vi "prediction bounds.vi"(6 "damping":dbl, 7 "amplitude":dbl, 8 "error in (no error)":errorcluster, 9 "Hours array":dbl[](array[numeric]), 10 "Previous Hours Array":dbl[](array[numeric]), 11 "Previous Data Array":dbl[](array[numeric])) -> (0 "error out":errorcluster, 2 "Lower Bound":cluster{"Hours array":dbl[], "P(A)":dbl[]}, 3 "Upper Bound":cluster{"Hours array":dbl[], "P(A)":dbl[]})   [LabVIEW 2014, in "Data Trends.lvlib"]
uses:
  Data Trends.lvlib
  <vilib>/Analysis/6fits.llb/Prediction Interval (Exp).vi
  <vilib>/Analysis/polynomials.llb/1D Polynomial Evaluation (DBL).vi
  <vilib>/Analysis/NI_AALPro.lvlib
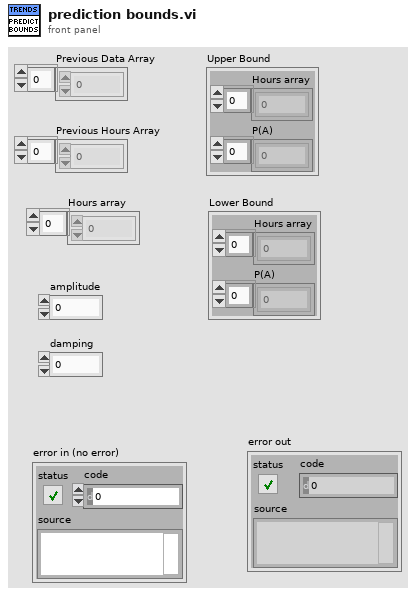
[diagram p1: front panel]
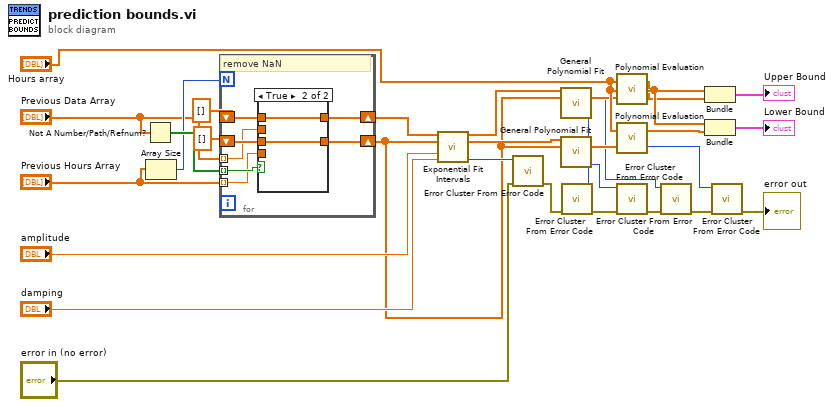
[diagram p0: block diagram]
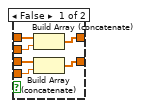
[diagram p2: hidden frame]
diagram:
  n1 = Not A Number/Path/Refnum?(number/path/refnum="Previous Data Array") -> (NaN/Path/Refnum?=w10:bool[])
  n2 = Array Size(array="Previous Hours Array") -> (size(s)=w9:i32)
  n3 = for {
    N: w9 -> [_]
    tunnel: w10 -> [w37] mode=indexing
    shift-right: [w36] -> w3
    shift-left: dbl[] [] -> [w35]
    shift-right: [w34] -> w6
    shift-left: dbl[] [] -> [w33]
    tunnel: "Previous Hours Array" -> [w32] mode=indexing
    tunnel: "Previous Data Array" -> [w31] mode=indexing
    # "remove NaN"
    n4 = case shown="True" w37 {
      tunnel: [w42 w45] -> w36
      tunnel: w35 -> [w43 w45]
      tunnel: [w41 w44] -> w34
      tunnel: w33 -> [w40 w44]
      tunnel: w32 -> [w39 _]
      tunnel: w31 -> [w38 _]
      frame False {
        n5 = Build Array (concatenate)(w40, w38) -> (w41:dbl[])
        n6 = Build Array (concatenate)(w43, w39) -> (w42:dbl[])
      }
      frame True {
      }
    }
  }
  n7 = call-poly <vilib>:"Exponential Fit Intervals.vi"("Y"=w6, "X"=w3, "amplitude"="amplitude", "damping"="damping") -> ("Upper Bound"=w26:dbl[], "Lower Bound"=w24:dbl[], "error"=w21:i32)  [unwired: 9 in]
  n8 = call <vilib>:"Error Cluster From Error Code.vi"("error in (no error)"="error in (no error)", "error code (0)"=w21) -> ("error out"=w19:errorcluster)  [unwired: 7 in]
  n9 = call <vilib>:"General Polynomial Fit.vi"("Y"=w26, "X"=w3) -> ("Polynomial Coefficients"=w28:dbl[], "error"=w16:i32)  [unwired: 10 in, 2 out]
  n10 = call <vilib>:"General Polynomial Fit.vi"("Y"=w24, "X"=w3) -> ("Polynomial Coefficients"=w25:dbl[], "error"=w15:i32)  [unwired: 10 in, 2 out]
  n11 = call <vilib>:"Error Cluster From Error Code.vi"("error in (no error)"=w19, "error code (0)"=w16) -> ("error out"=w18:errorcluster)  [unwired: 7 in]
  n12 = call-poly <vilib>:"Polynomial Evaluation.vi"("P(x)"=w28, "A"="Hours array") -> ("error"=w14:i32, "P(A)"=w2:dbl[])
  n13 = call-poly <vilib>:"Polynomial Evaluation.vi"("P(x)"=w25, "A"="Hours array") -> ("error"=w12:i32, "P(A)"=w1:dbl[])
  n14 = call <vilib>:"Error Cluster From Error Code.vi"("error in (no error)"=w18, "error code (0)"=w15) -> ("error out"=w17:errorcluster)  [unwired: 7 in]
  n15 = call <vilib>:"Error Cluster From Error Code.vi"("error in (no error)"=w17, "error code (0)"=w14) -> ("error out"=w13:errorcluster)  [unwired: 7 in]
  n16 = Bundle("Hours array"="Hours array", "P(A)"=w2) -> (→"Upper Bound":cluster{"Hours array":dbl[], "P(A)":dbl[]})  [unwired: 1 in]
  n17 = Bundle("Hours array"="Hours array", "P(A)"=w1) -> (→"Lower Bound":cluster{"Hours array":dbl[], "P(A)":dbl[]})  [unwired: 1 in]
  n18 = call <vilib>:"Error Cluster From Error Code.vi"("error in (no error)"=w13, "error code (0)"=w12) -> ("error out"=→"error out":errorcluster)  [unwired: 7 in]
